vi "Create-Delete Directory.vi"(5 "Username":string, 6 "Password":string, 7 "Address":string, 8 "Error In":errorcluster) -> (0 "Error Out":errorcluster)   [LabVIEW 2018, in "Tests.lvlib" / "SFTP.lvlib"]
uses:
  SFTP.lvlib
  src/Toolkit/API/SFTP File/API/Typedefs/Flags.ctl
  src/Toolkit/API/SFTP Attributes/API/Typedefs/File Types.ctl
  src/Toolkit/API/SFTP Attributes/SFTP Attributes.lvclass/SFTP Attributes.ctl
  src/Toolkit/API/SSH/SSH.lvclass/SSH.ctl
  src/Toolkit/API/SSH/Utility/Read Shared Library.vi
  src/Toolkit/API/SFTP Attributes/Support/Create from SFTP File.vi
  src/Toolkit/Support/Check Status.vi
  src/Toolkit/API/SFTP Attributes/Support/Destroy to SFTP File.vi
  <vilib>/addons/_JKI Toolkits/Caraya/classes/Test/Test.lvclass
  <vilib>/addons/_JKI Toolkits/Caraya/classes/Assert/Assert.lvclass
  src/Toolkit/API/SFTP/SFTP.lvclass
  src/Toolkit/API/SFTP File/SFTP File.lvclass
  src/Toolkit/API/SFTP Attributes/SFTP Attributes.lvclass
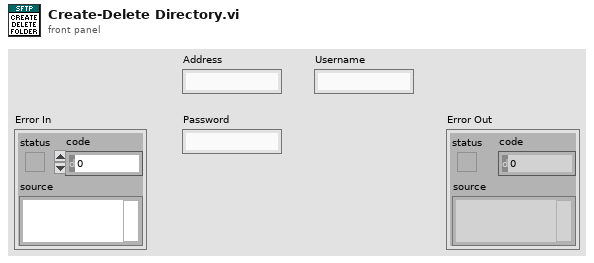
[diagram p1: front panel]
types:
  T1 = typedef "Toolkit.lvlib/SFTP Attributes.lvclass/File Types.ctl" = u32
  T2 = typedef "Toolkit.lvlib/SFTP File.lvclass/Flags.ctl" = cluster{"Read":bool, "Write":bool, "Append":bool, "Create":bool, "Truncate":bool, "Exclude":bool}
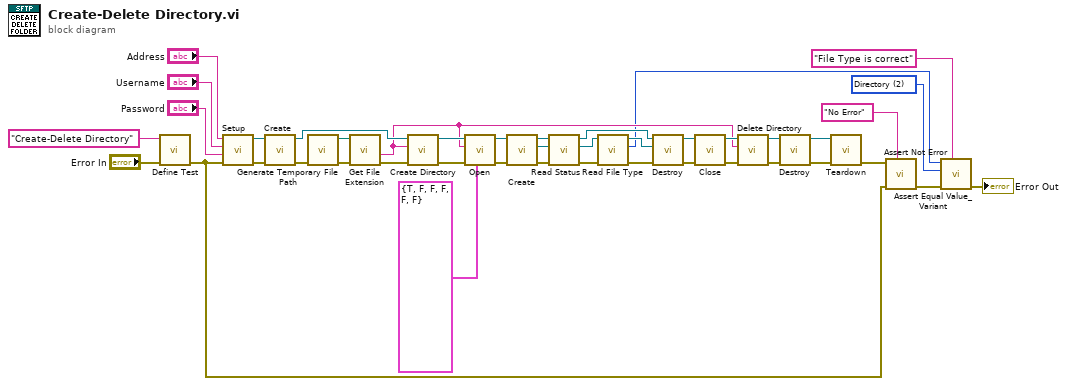
[diagram p0: block diagram]
diagram:
  w1 = T1 2 items=["Regular"=1, "Directory"=2, "Symbolic Link"=3, "Special"=4, "Unknown"=5, "Socket"=6, "Character Device"=7, "Block Device"=8, "FIFO"=9] ("File Type")
  n1 = call <vilib>:"Define Test.vi"("error in (no error)"="Error In", "Label (VI Title)"="Create-Delete Directory") -> ("error out"=w37:errorcluster)  [unwired: 9 in]
  n2 = call "Setup.vi"("Error In"=w37, "Password"="Password", "Username"="Username", "Address"="Address") -> ("Error Out"=w38:errorcluster, "Sesssion"=w33:refnum<class "Session.lvclass">)  [unwired: 6 in]
  n3 = call "Create.vi"("Error In"=w38, "Session"=w33) -> ("Error Out"=w29:errorcluster, "SFTP"=w25:refnum<class "SFTP.lvclass">)  [unwired: 8 in]
  n4 = call <vilib>:"Generate Temporary File Path.vi"("error in (no error)"=w29) -> ("error out"=w27:errorcluster, "Unique Temporary File Path"=w28:path)  [unwired: 9 in]
  n5 = call <vilib>:"Get File Extension.vi"("error in (no error)"=w27, "file"=w28) -> ("error out"=w26:errorcluster, "filename without extension"=w7:string)  [unwired: 5 in, 3 out]
  n6 = call "Create Directory.vi"("Error In"=w26, "Remote Path"=w7, "SFTP In"=w25) -> ("Error Out"=w22:errorcluster, "SFTP Out"=w21:refnum<class "SFTP.lvclass">)  [unwired: 7 in]
  n7 = call "Open.vi"("Flags"=T2 {"Read"=TRUE, "Write"=FALSE, "Append"=FALSE, "Create"=FALSE, "Truncate"=FALSE, "Exclude"=FALSE}, "Error In"=w22, "Remote Path"=w7, "SFTP"=w21) -> ("Error Out"=w15:errorcluster, "SFTP File"=w20:refnum<class "SFTP File.lvclass">)  [unwired: 6 in]
  n8 = call-poly "Create.vi"("Error In"=w15, "SFTP File In"=w20) -> ("Error Out"=w14:errorcluster, "SFTP Attributes"=w18:refnum<class "SFTP Attributes.lvclass">, "SFTP File Out"=w19:refnum<class "SFTP File.lvclass">)  [unwired: 7 in]
  n9 = call "Read Status.vi"("Error In"=w14, "Attributes In"=w18, "SFTP File In"=w19) -> ("Error Out"=w13:errorcluster, "Attributes Out"=w16:refnum<class "SFTP Attributes.lvclass">, "SFTP File Out"=w17:refnum<class "SFTP File.lvclass">)  [unwired: 6 in]
  n10 = call "Read File Type.vi"("Error In"=w13, "SFTP Attributes In"=w16) -> ("Error Out"=w12:errorcluster, "File Type"=w3:T1, "SFTP Attribute Out"=w5:refnum<class "SFTP Attributes.lvclass">)  [unwired: 7 in]
  n11 = call-poly "Destroy.vi"("Error In"=w12, "SFTP Attributes"=w5, "SFTP File In"=w17) -> ("Error Out"=w11:errorcluster, "SFTP File Out"=w9:refnum<class "SFTP File.lvclass">)  [unwired: 7 in]
  n12 = call "Close.vi"("Error In"=w11, "SFTP File"=w9) -> ("Error Out"=w10:errorcluster, "SFTP"=w8:refnum<class "SFTP.lvclass">)  [unwired: 7 in, 1 out]
  n13 = call "Delete Directory.vi"("Error In"=w10, "Remote Path"=w7, "SFTP In"=w8) -> ("Error Out"=w24:errorcluster, "SFTP Out"=w23:refnum<class "SFTP.lvclass">)  [unwired: 7 in]
  n14 = call "Destroy.vi"("Error In"=w24, "SFTP"=w23) -> ("Error Out"=w32:errorcluster, "Session"=w30:refnum<class "Session.lvclass">)  [unwired: 8 in]
  n15 = call "Teardown.vi"("Error In"=w32, "Session"=w30) -> ("Error Out"=w31:errorcluster)  [unwired: 9 in]
  n16 = call <vilib>:"Assert Not Error.vi"("Label"="No Error", "error in (no error)"=w37, "Not Error?"=w31) -> ("error out"=w39:errorcluster)  [unwired: 8 in]
  n17 = call <vilib>:"Assert Equal Value_Variant.vi"("Label"="File Type is correct", "error in (no error)"=w39, "Y"=w1, "X"=w3) -> ("error out"=→"Error Out":errorcluster)  [unwired: 7 in]
